vi "Comparador.vi"() -> ()   [LabVIEW 2014]
uses:
  <vilib>/Analysis/2dsp.llb/Real FFT.vi
  <vilib>/Analysis/2dsp.llb/Inverse Complex FFT.vi
  <vilib>/Utility/file.llb/Read From Spreadsheet File (string).vi
  <vilib>/Analysis/NI_AALPro.lvlib
panel:
  out "Curva de Engranes":dbl[][](graph)
  out "Transductores":string[][](table)
  out "Resultado Z1:":dbl format="%#_16g"
  # "Tabla de Transductores"
  # "El programa carga el archivo que genera\nMatlab donde el mismo contiene los \nvalores de la funcion original y los \ncalculados por este mismo.\n\nCurva Roja: Es la curva generada por \nLabView con los mismo algoritmos del \nmodulo matemático.\n\nCurva Azul: Es la curva generada por \nMatlab desde el Script \"ResultadoZ1.m\".\n\nCurva Verde: Es la diferencia entre \nla curva de LabView y la de Matlab."
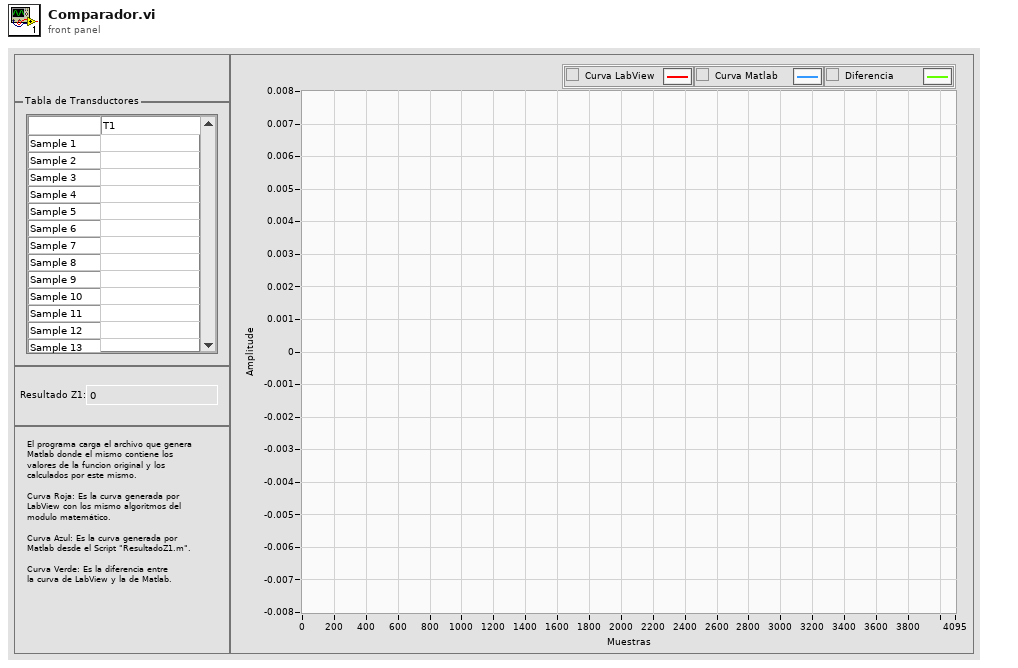
[diagram p1: front panel]
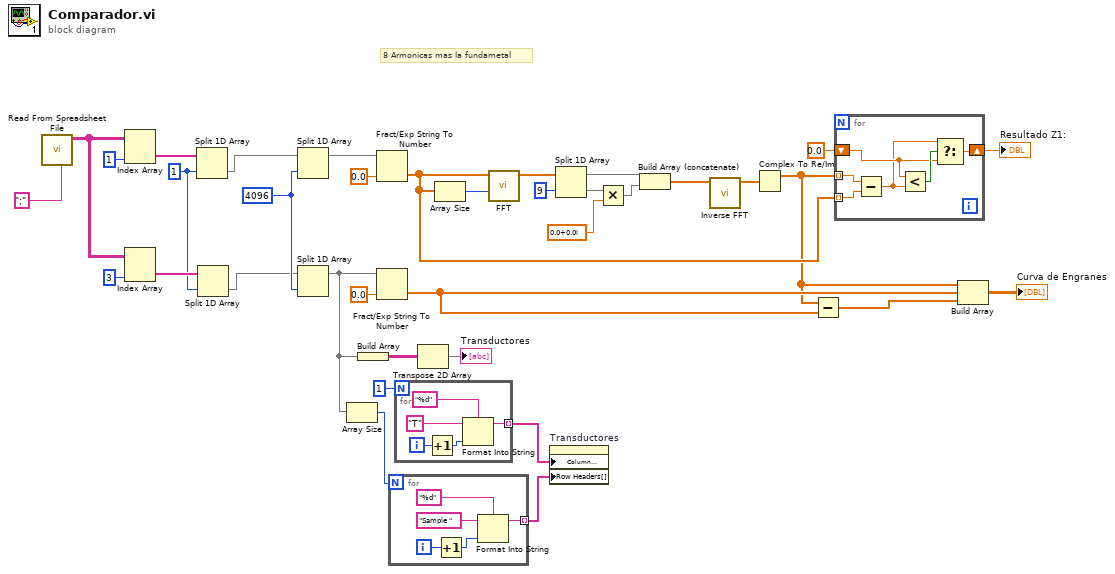
[diagram p0: block diagram]
diagram:
  w2 = 1 ("disabled index (col)")
  w15 = 4096 ("index")
  # "8 Armonicas mas la fundametal"
  n1 = call-poly <vilib>:"Read From Spreadsheet File.vi"("delimiter (\\t)"=";" ("delimiter (\\t)")) -> ("all rows"=w11:string[][])  [unwired: 6 in, 4 out]
  n2 = Index Array(array=w11, index (col)=1 ("disabled index (col)")) -> (element=w3:string[])  [unwired: 1 in]
  n3 = Index Array(array=w11, index (col)=3 ("disabled index (col)")) -> (element=w6:string[])  [unwired: 1 in]
  n4 = Split 1D Array(array=w3, index=w2) -> (second subarray=w4:string[])  [unwired: 1 out]
  n5 = Split 1D Array(array=w6, index=w2) -> (second subarray=w5:string[])  [unwired: 1 out]
  n6 = Split 1D Array(array=w4, index=w15) -> (first subarray=w16:string[])  [unwired: 1 out]
  n7 = Split 1D Array(array=w5, index=w15) -> (first subarray=w1:string[])  [unwired: 1 out]
  n8 = Array Size(array=w1) -> (size(s)=w10:i32)
  n9 = Build Array(w1) -> (w8:string[][])
  n10 = Fract/Exp String To Number(string=w16, default (0 dbl)=0.0 ("default (0 DBL)")) -> (number=w25:dbl[])  [unwired: 2 in, 1 out]
  n11 = Fract/Exp String To Number(string=w1, default (0 dbl)=0.0 ("default (0 DBL)")) -> (number=w20:dbl[])  [unwired: 2 in, 1 out]
  n12 = for {
    N: w10 -> [_]
    tunnel: [w41] -> w13 mode=indexing
    i -> [w38]
    n13 = Increment(x=w38) -> (x+1=w37:i32)
    n14 = Format Into String(format string="%d", initial string="Sample ", w37) -> (resulting string=w41:string)  [unwired: 1 in, 1 out]
  }
  n15 = for {
    N: 1 -> [_]
    tunnel: [w46] -> w12 mode=indexing
    i -> [w43]
    n16 = Increment(x=w43) -> (x+1=w42:i32)
    n17 = Format Into String(format string="%d", initial string="T", w42) -> (resulting string=w46:string)  [unwired: 1 in, 1 out]
  }
  n18 = Transpose 2D Array(2D array=w8) -> (transposed array=→"Transductores":string[][])
  n19 = Array Size(array=w25) -> (size(s)=w26:i32)
  n20 = call-poly <vilib>:"FFT.vi"("FFT size"=w26, "X"=w25) -> ("FFT {X}"=w34:cdb[])  [unwired: 8 in, 1 out]
  n21 = property on="Transductores" class="Tbl (strict)"("Column Headers[]"=w12, "Row Headers[]"=w13) -> ()  [unwired: 2 in, 2 out]
  n22 = Split 1D Array(array=w34, index=9) -> (first subarray=w31:cdb[], second subarray=w32:cdb[])
  n23 = Multiply(x=w32, y=cdb 0.0+0.0i) -> (x*y=w30:cdb[])
  n24 = Build Array (concatenate)(w31, w30) -> (w28:cdb[])
  n25 = call-poly <vilib>:"Inverse FFT.vi"("FFT {X}"=w28) -> ("X"=w18:cdb[])  [unwired: 9 in, 1 out]
  n26 = Complex To Re/Im(x + iy=w18) -> (x=w17:dbl[])  [unwired: 1 out]
  n27 = Subtract(x=w17, y=w20) -> (x-y=w19:dbl[])
  n28 = for {
    tunnel: w25 -> [w51] mode=indexing
    tunnel: w17 -> [w52] mode=indexing
    shift-right: [w47] -> w24
    shift-left: 0.0 -> [w49]
    n29 = Subtract(x=w52, y=w51) -> (x-y=w48:dbl)
    n30 = Less?(x=w49, y=w48) -> (x < y?=w50:bool)
    n31 = Select(t=w48, s=w50, f=w49) -> (s? t:f=w47:dbl)
  }
  "Resultado Z1:" <- w24
  n32 = Build Array(w17, w20, w19) -> (→"Curva de Engranes":dbl[][])
